vi "FTW-CodeGen-Prototype.vi"(0 "REPLACE_FTW Actor Connector":T1, 5 "ADAPT_Request":string, 7 "ADAPT_Response Type and Defaults":string, 9 "REPLACE_Timeout":i32=100 format="%dmsec", 11 "REPLACE_error in":errorcluster) -> (4 "REPLACE_FTW Actor Connector out":T1, 8 "ADAPT_Response":string, 10 "REPLACE_Roundtrip Time":dbl format="%.4psec", 15 "REPLACE_error out":errorcluster)   [LabVIEW 2015, in "FTW-Actor-Ask.xnode"]
uses:
  FTW-Actor-Ask.xnode
  src/core/type/FTW-Type-Actor-Connector.ctl
  src/error/FTW-ERR-ThrowError.vi
  src/reflection/FTW-Reflection-Type.vi
  src/error/FTW-ERR-NoErrorConstant.vi
  src/error/FTW-ERR-CallChain.vi
  src/string/FTW-STR-ReplaceWhitespace.vi
  src/reflection/FTW-Reflection-Array.vi
  src/reflection/FTW-Reflection-FTWObject.vi
  src/string/FTW-STR-Array-Delimit.vi
  src/json/core/FTW-JSON-Core-EncodingFlags.vi
  json/fetch/FTW-JSON-Core-GetFlattenedValue.vi
  FTW-JSON-Fetch.xnode
panel:
  # "Inputs"
  # "Outputs"
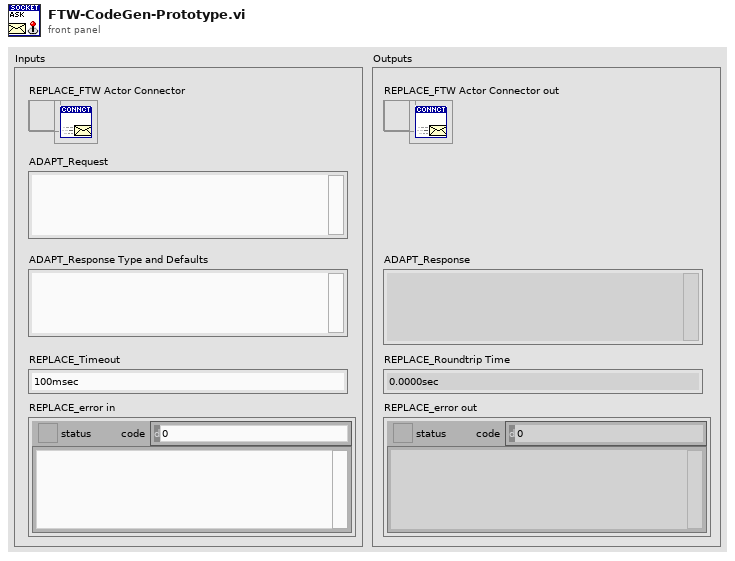
[diagram p1: front panel]
types:
  T1 = typedef "FTW-Type-Actor-Connector.ctl" = refnum<data-value>
  T2 = cluster{"FTW-CodeGen-Type":enum16{"FTW-Actor-Connector"}, "Socket":i64}
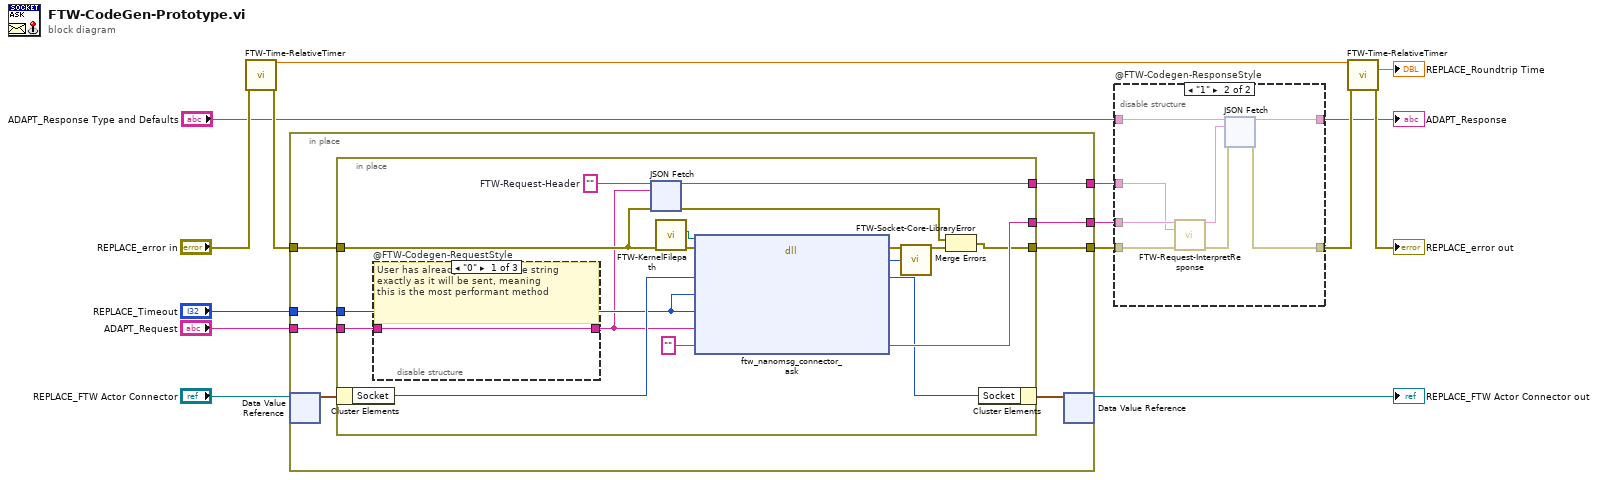
[diagram p0: block diagram]
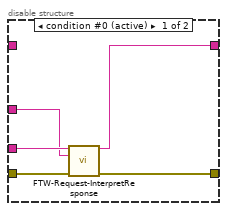
[diagram p2: hidden frame]
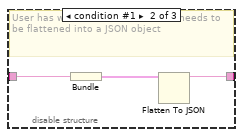
[diagram p3: hidden frame]
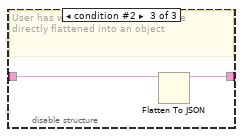
[diagram p4: hidden frame]
diagram:
  n1 = call "FTW-Time-RelativeTimer.vi"("error in"="REPLACE_error in") -> ("Current Timer Value"=w9:dbl, "error out"=w10:errorcluster)  [unwired: 12 in, 1 out]
  n2 = in-place {
    in-place-border: w10 -> [w23]
    in-place-border: [w22] -> w6
    in-place-border: [w21] -> w5
    in-place-border: "REPLACE_Timeout" -> [w20]
    in-place-border: "ADAPT_Request" -> [w19]
    in-place-border: [w16] -> w4
    n3 = in-place-dvr #1("REPLACE_FTW Actor Connector") -> (w18:T2)  [unwired: 1 out]
    n4 = in-place {
      in-place-border: w23 -> [w32]
      in-place-border: [w30] -> w22
      in-place-border: [w39] -> w21
      in-place-border: w20 -> [w27]
      in-place-border: w19 -> [w28]
      in-place-border: [w29] -> w16
      w26 = ""  # FTW-Request-Header
      n5 = in-place-cluster #2(w18) -> ("Socket"=w36:i64)
      n6 = disable-structure "@FTW-Codegen-RequestStyle" shown="\"0\"" {
        disable-tunnel: w28 -> [w41 w44 w46]
        disable-tunnel: [w41 w43 w45] -> w25
        frame condition #0 (active) {
          # "User has already formatted the string\nexactly as it will be sent, meaning\nthis is the most performant method"
        }
        frame condition #1 {
          # "User has wired a scalar value that needs to\nbe flattened into a JSON object"
          n7 = Bundle("ADAPT_Request"=w44) -> (w42:cluster{"ADAPT_Request":string})  [unwired: 1 in]
          n8 = Flatten To JSON(anything=w42) -> (JSON string=w43:string)  [unwired: 2 in, 1 out]
        }
        frame condition #2 {
          # "User has wired a cluster that can be\ndirectly flattened into an object"
          n9 = Flatten To JSON(anything=w46) -> (JSON string=w45:string)  [unwired: 2 in, 1 out]
        }
      }
      n10 = xnode "JSON Fetch"("Type and Defaults"=w26, "JSON String"=w25, "error in"=w32) -> ("Values"=w29:string, "error out"=w24:errorcluster)  [unwired: 1 in]
      n11 = call "FTW-KernelFilepath.vi"("error in"=w32) -> ("error out"=w34:errorcluster, "Library Filepath"=w33:path)  [unwired: 8 in, 1 out]
      n12 = dll-call lib="?" fn="ftw_nanomsg_connector_ask"(path in=w33, error in=w34, "Socket Handle"=w36, "Send Timeout"=w27, "Recv Timeout"=w27, "Request"=w25, "Response"="") -> (error out=w40:errorcluster, "Return Value"=w38:i64, "Socket Handle"=w35:i64, "Response"=w39:string)  [unwired: 4 in, 1 out]
      n13 = call "FTW-Socket-Core-LibraryError.vi"("error in"=w40, "Return Value"=w38) -> ("error out"=w31:errorcluster)  [unwired: 13 in]
      n14 = Merge Errors(w24, w31) -> (w30:errorcluster)
      n15 = in-place-cluster #2("Socket"=w35) -> (w17:T2)
    }
    n16 = in-place-dvr #1(w17) -> (→"REPLACE_FTW Actor Connector out":T1)  [unwired: 1 out]
  }
  n17 = disable-structure "@FTW-Codegen-ResponseStyle" shown="\"1\"" {
    disable-tunnel: w6 -> [w117 w125]
    disable-tunnel: w5 -> [w116 w124]
    disable-tunnel: w4 -> [w115 w123]
    disable-tunnel: "ADAPT_Response Type and Defaults" -> [_ w122]
    disable-tunnel: [w113 w120] -> w2
    disable-tunnel: [w114 w119] -> w1
    frame condition #0 (active) {
      n18 = call "FTW-Request-InterpretResponse.vi"("Raw Request"=w116, "Request Header"=w115, "error in"=w117) -> ("JSON Response"=w114:string, "error out"=w113:errorcluster)  [unwired: 11 in]
    }
    frame condition #1 {
      n19 = call "FTW-Request-InterpretResponse.vi"("Raw Request"=w124, "Request Header"=w123, "error in"=w125) -> ("JSON Response"=w118:string, "error out"=w121:errorcluster)  [unwired: 11 in]
      n20 = xnode "JSON Fetch"("Type and Defaults"=w122, "JSON String"=w118, "error in"=w121) -> ("Values"=w119:string, "error out"=w120:errorcluster)  [unwired: 1 in]
    }
  }
  "ADAPT_Response" <- w1
  n21 = call "FTW-Time-RelativeTimer.vi"("Previous Timer Value"=w9, "error in"=w2) -> ("Elapsed Time"=→"REPLACE_Roundtrip Time":dbl, "error out"=→"REPLACE_error out":errorcluster)  [unwired: 11 in, 1 out]
